vi "DDS Re-initialize One Channel.vi"(4 "channel number (1)":u8=1 min=1 max=4 step=1, 6 "error in (no error)":errorcluster, 9 "DDS ref in":T1) -> (0 "error out":errorcluster, 3 "DDS ref out":T1)   [LabVIEW 2013, in "DDS.lvlib"]
doc: "Resets and re-initializes the AD9910 registers for the given channel."
uses:
  DDS.lvlib
  Controls/DDS Box Device Reference.ctl
  <vilib>/ni845x/ni845x.llb/ni845xControl.ctl
  Controls/AD9910 registers.ctl
  <vilib>/ni845x/ni845x.llb/NI-845x SPI Script Ms Delay.vi
panel:
  out "CFR3":u8[](array[numeric])
  out "CFR1":u8[](array[numeric])
  out "CFR2":u8[](array[numeric])
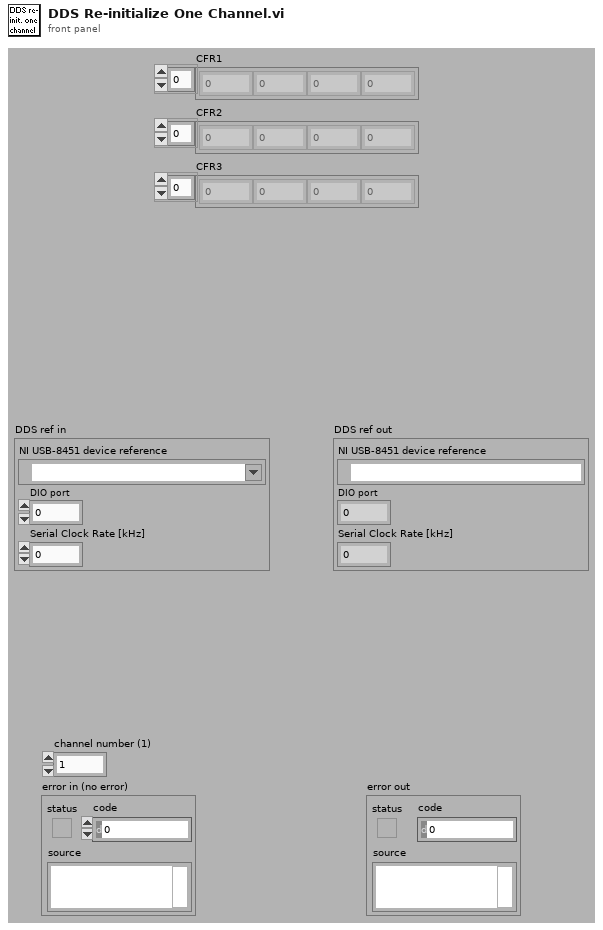
[diagram p1: front panel]
types:
  T1 = typedef "DDS.lvlib/DDS Box Device Reference.ctl" = cluster{"NI USB-8451 device reference":T2, "DIO port":u8, "Serial Clock Rate [kHz]":u16}
  T2 = typedef "ni845xControl.ctl" = refnum<k21>
  T3 = typedef "ni845xSpiScriptControl.ctl" = refnum<k20>
  T4 = typedef "DDS.lvlib/AD9910 registers.ctl" = enum16{"CFR1", "CFR2", "CFR3", "Auxiliary DAC Control", "I/0 Update Rate", "Frequency Tuning Word", "Phase Offset Word", "Amplitude Scale Factor", "Multichip Sync", "Digital Ramp Limit", "Digital Ramp Step Size", "Digital Ramp Rate", "Single Tone Profile 0", "Single Tone Profile 1", "Single Tone Profile 2", "Single Tone Profile 3", "Single Tone Profile 4", "Single Tone Profile 5", "Single Tone Profile 6", "Single Tone Profile 7", "RAM Profile 0", "RAM Profile 1", "RAM Profile 2", "RAM Profile 3", "RAM Profile 4", "RAM Profile 5", "RAM Profile 6", "RAM Profile 7", "RAM"}
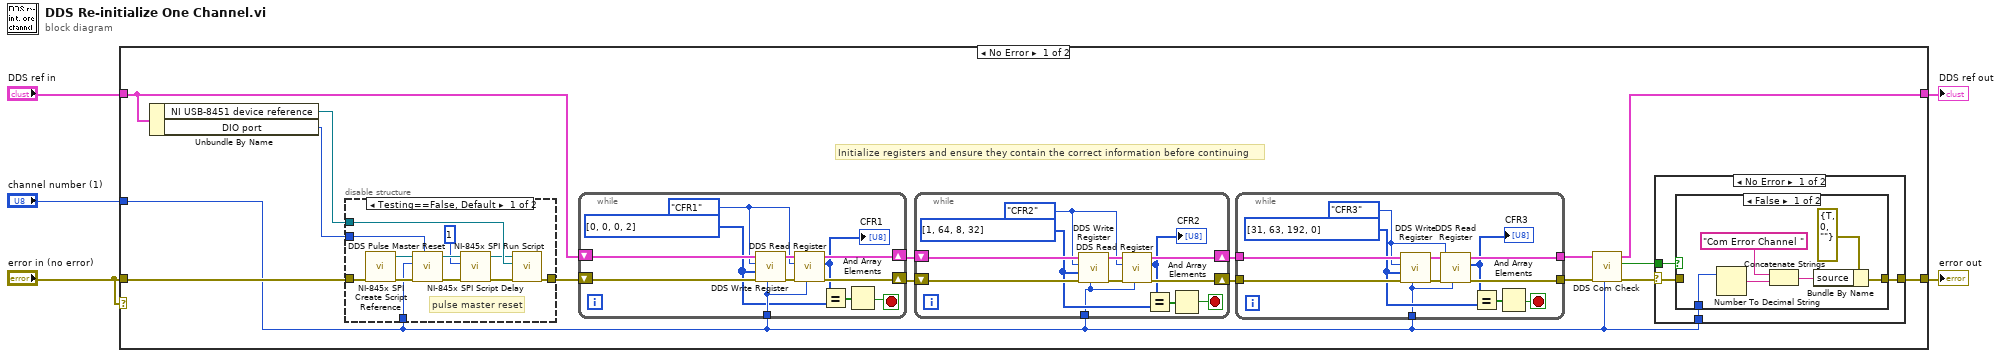
[diagram p0: block diagram]
diagram:
  n1 = case shown="No Error" "error in (no error)" {
    tunnel: "error in (no error)" -> [w20 w84]
    tunnel: [w13 w83] -> w5
    tunnel: [w16 w84] -> w4
    tunnel: "DDS ref in" -> [w19 w83]
    tunnel: "channel number (1)" -> [w10 _]
    frame No Error {
      # "Initialize registers and ensure they contain the correct information before continuing"
      n2 = Unbundle By Name(w19) -> ("NI USB-8451 device reference"=w18:T2, "DIO port"=w17:u8)
      n3 = disable-structure shown="Testing==False, Default" {
        disable-tunnel: w20 -> [w81 w82]
        disable-tunnel: [w79 w82] -> w21
        disable-tunnel: w17 -> [w77 _]
        disable-tunnel: w18 -> [w76 _]
        disable-tunnel: w10 -> [w70 _]
        frame condition #0 (active) {
          # "pulse master reset"
          n4 = call <vilib>:"NI-845x SPI Create Script Reference.vi"("error in (no error)"=w81) -> ("error out"=w80:errorcluster, "spi script reference"=w78:T3)  [unwired: 9 in]
          n5 = call "DDS Pulse Master Reset.vi"("port number (0)"=w77, "error in (no error)"=w80, "channel number (1)"=w70, "spi script reference in"=w78) -> ("error out"=w74:errorcluster, "spi script reference out"=w75:T3)  [unwired: 6 in]
          n6 = call-poly <vilib>:"NI-845x SPI Script Delay.vi"("error in (no error)"=w74, "delay in milliseconds (0)"=u8 1, "spi script reference in"=w75) -> ("error out"=w73:errorcluster, "spi script reference out"=w72:T3)  [unwired: 7 in]
          n7 = call <vilib>:"NI-845x SPI Run Script.vi"("error in (no error)"=w73, "device reference in"=w76, "spi script reference in"=w72) -> ("error out"=w79:errorcluster)  [unwired: 6 in, 2 out]
        }
        frame condition #1 {
        }
      }
      n8 = while {
        tunnel: w10 -> [w50]
        shift-right: [w52] -> w11
        shift-left: w19 -> [w56]
        shift-right: [w53] -> w12
        shift-left: w21 -> [w57]
        stop <- w46 stop-if-true
        w48 = u8[] [0, 0, 0, 2] ("Write Data")
        w51 = AD9910_registers."CFR1" ("Register")
        n9 = call "DDS Write Register.vi"("channel number (1)"=w50, "error in (no error)"=w57, "Write Data"=w48, "Register"=w51, "DDS ref in"=w56) -> ("error out"=w54:errorcluster, "DDS ref out"=w55:T1)  [unwired: 4 in, 1 out]
        n10 = call "DDS Read Register.vi"("channel number (1)"=w50, "error in (no error)"=w54, "Register"=w51, "DDS ref in"=w55) -> ("error out"=w53:errorcluster, "Read data"=w49:u8[], "DDS ref out"=w52:T1)  [unwired: 5 in]
        "CFR1" <- w49
        n11 = Equal?(x=w49, y=w48) -> (x = y?=w47:bool[])
        n12 = And Array Elements(Boolean array=w47) -> (logical AND=w46:bool)
      }
      n13 = while {
        tunnel: w10 -> [w35]
        shift-right: [w41] -> w9
        shift-left: w12 -> [w45]
        shift-right: [w40] -> w8
        shift-left: w11 -> [w44]
        stop <- w38 stop-if-true
        w36 = u8[] [1, 64, 8, 32] ("Write Data")
        w34 = AD9910_registers."CFR2" ("Register")
        n14 = call "DDS Write Register.vi"("channel number (1)"=w35, "error in (no error)"=w45, "Write Data"=w36, "Register"=w34, "DDS ref in"=w44) -> ("error out"=w42:errorcluster, "DDS ref out"=w43:T1)  [unwired: 4 in, 1 out]
        n15 = call "DDS Read Register.vi"("channel number (1)"=w35, "error in (no error)"=w42, "Register"=w34, "DDS ref in"=w43) -> ("error out"=w41:errorcluster, "Read data"=w37:u8[], "DDS ref out"=w40:T1)  [unwired: 5 in]
        "CFR2" <- w37
        n16 = Equal?(x=w37, y=w36) -> (x = y?=w39:bool[])
        n17 = And Array Elements(Boolean array=w39) -> (logical AND=w38:bool)
      }
      n18 = while {
        tunnel: w10 -> [w22]
        tunnel: w9 -> [w33]
        tunnel: w8 -> [w32]
        tunnel: [w29] -> w7
        tunnel: [w28] -> w6
        stop <- w23 stop-if-true
        w24 = u8[] [31, 63, 192, 0] ("Write Data")
        w26 = AD9910_registers."CFR3" ("Register")
        n19 = call "DDS Write Register.vi"("channel number (1)"=w22, "error in (no error)"=w33, "Write Data"=w24, "Register"=w26, "DDS ref in"=w32) -> ("error out"=w30:errorcluster, "DDS ref out"=w31:T1)  [unwired: 4 in, 1 out]
        n20 = call "DDS Read Register.vi"("channel number (1)"=w22, "error in (no error)"=w30, "Register"=w26, "DDS ref in"=w31) -> ("error out"=w29:errorcluster, "Read data"=w25:u8[], "DDS ref out"=w28:T1)  [unwired: 5 in]
        "CFR3" <- w25
        n21 = Equal?(x=w25, y=w24) -> (x = y?=w27:bool[])
        n22 = And Array Elements(Boolean array=w27) -> (logical AND=w23:bool)
      }
      n23 = call "DDS Com Check.vi"("channel number (1)"=w10, "error in (no error)"=w7, "DDS ref in"=w6) -> ("error out"=w15:errorcluster, "Passed?"=w14:bool, "DDS ref out"=w13:T1)  [unwired: 4 in]
      n24 = case shown="No Error" w15 {
        selector: w15 -> [w58 w69]
        tunnel: w14 -> [w61 _]
        tunnel: [w60 w69] -> w16
        tunnel: w10 -> [w59 _]
        frame No Error {
          n25 = case shown="False" w61 {
            tunnel: [w66 w68] -> w60
            tunnel: w59 -> [w62 _]
            tunnel: w58 -> [_ w68]
            frame False {
              n26 = Number To Decimal String(number=w62) -> (decimal integer string=w63:string)  [unwired: 1 in]
              n27 = Concatenate Strings("Com Error Channel " ("source"), w63) -> (w64:string)
              n28 = Bundle By Name(cluster=errorcluster {"status"=TRUE, "code"=0, "source"=""} ("error out"), "source"=w64) -> (w66:errorcluster)
            }
            frame True {
            }
          }
        }
        frame Error {
        }
      }
    }
    frame Error {
    }
  }
  "DDS ref out" <- w5
  "error out" <- w4
